vi "Get Key Value (Single).vi"(5 "Key name":string, 6 "Default value":sgl, 7 "Section name":string, 8 "error in (no error)":errorcluster, 11 "Carya Config in":refnum<class "Carya Config.lvclass">) -> (0 "error out":errorcluster, 1 "Found?":bool, 2 "Value":sgl format="%.2f", 3 "Carya Config out":refnum<class "Carya Config.lvclass">)   [LabVIEW 2013, in "Carya Config.lvclass"]
doc: "Copyright 2018, Carya Automatisering, Wiebe Walstra."
uses:
  Carya Config.lvclass
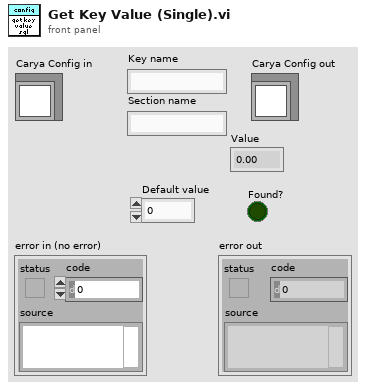
[diagram p1: front panel]
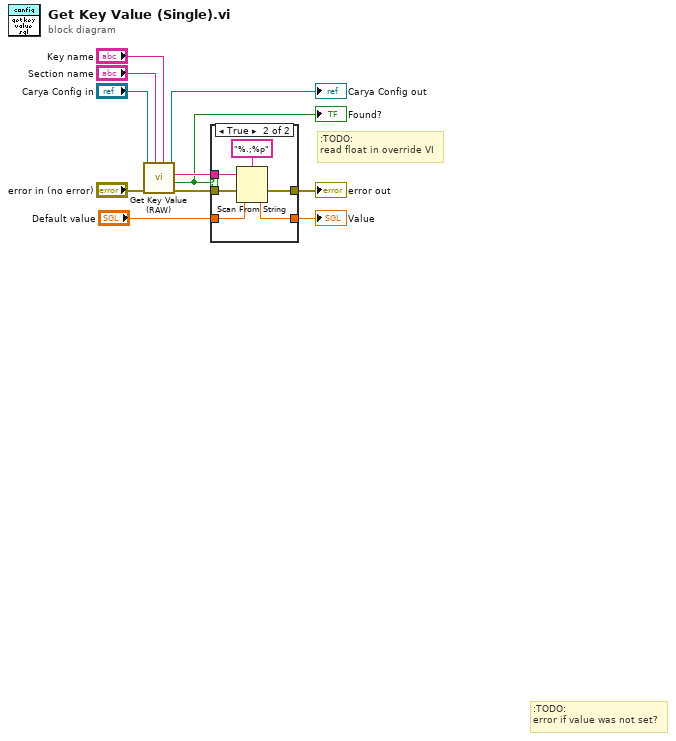
[diagram p0: block diagram]
diagram:
  # ":TODO:\nread float in override VI"
  # ":TODO:\nerror if value was not set?"
  n1 = call-dynamic "Get Key Value (RAW).vi"("Key name"="Key name", "Section name"="Section name", "error in (no error)"="error in (no error)", "Carya Config in"="Carya Config in") -> ("error out"=w10:errorcluster, "Found?"=w2:bool, "Value"=w4:string, "Carya Config out"=→"Carya Config out":refnum<class "Carya Config.lvclass">)  [unwired: 4 in]
  "Found?" <- w2
  n2 = case shown="True" w2 {
    tunnel: w10 -> [w12 w19]
    tunnel: [w12 w18] -> w5
    tunnel: w4 -> [_ w17]
    tunnel: "Default value" -> [w13 w16]
    tunnel: [w13 w15] -> w1
    frame False {
    }
    frame True {
      n3 = Scan From String(format string="%.;%p", input string=w17, error in=w19, default 1=w16) -> (error out=w18:errorcluster, output 1=w15:sgl)  [unwired: 1 in, 2 out]
    }
  }
  "error out" <- w5
  "Value" <- w1
